vi "GUNSC_test2.vi"() -> ()   [LabVIEW 2014]
uses:
  ctest/libmap.so
  Common/Clib/lib/libmem.so.20
  expglobal.vi
  flags.vi
panel:
  in  "writekey command":string
  in  "send unsc":bool
  in  "send geom":bool
  in  "Geometry command":string
  in  "new unscrambled image":path=path "/home/ArcVIEW/Modules/GUNSC/test/ctest/test"
  in  "multiple extensions":bool=TRUE
  in  "ReadModes":u16(ring)
  in  "FPA name":string="P60"
  in  "error in (no error)":errorcluster
  in  "naxis":i32
  in  "bitpix":i32
  in  "nrows":i32
  in  "ncols":i32
  in  "scramble image on disk":path=path "/home/ArcVIEW/Modules/GUNSC/test/ctest/scr.fits"
  in  "stop":bool
  in  "Pieces":u16=1 min=1
  in  "send":bool
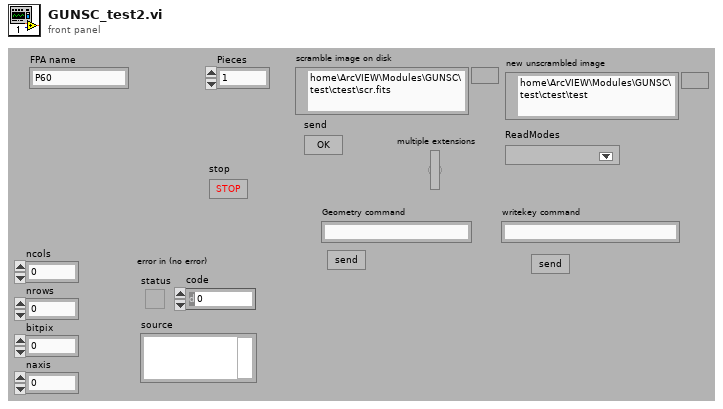
[diagram p1: front panel]
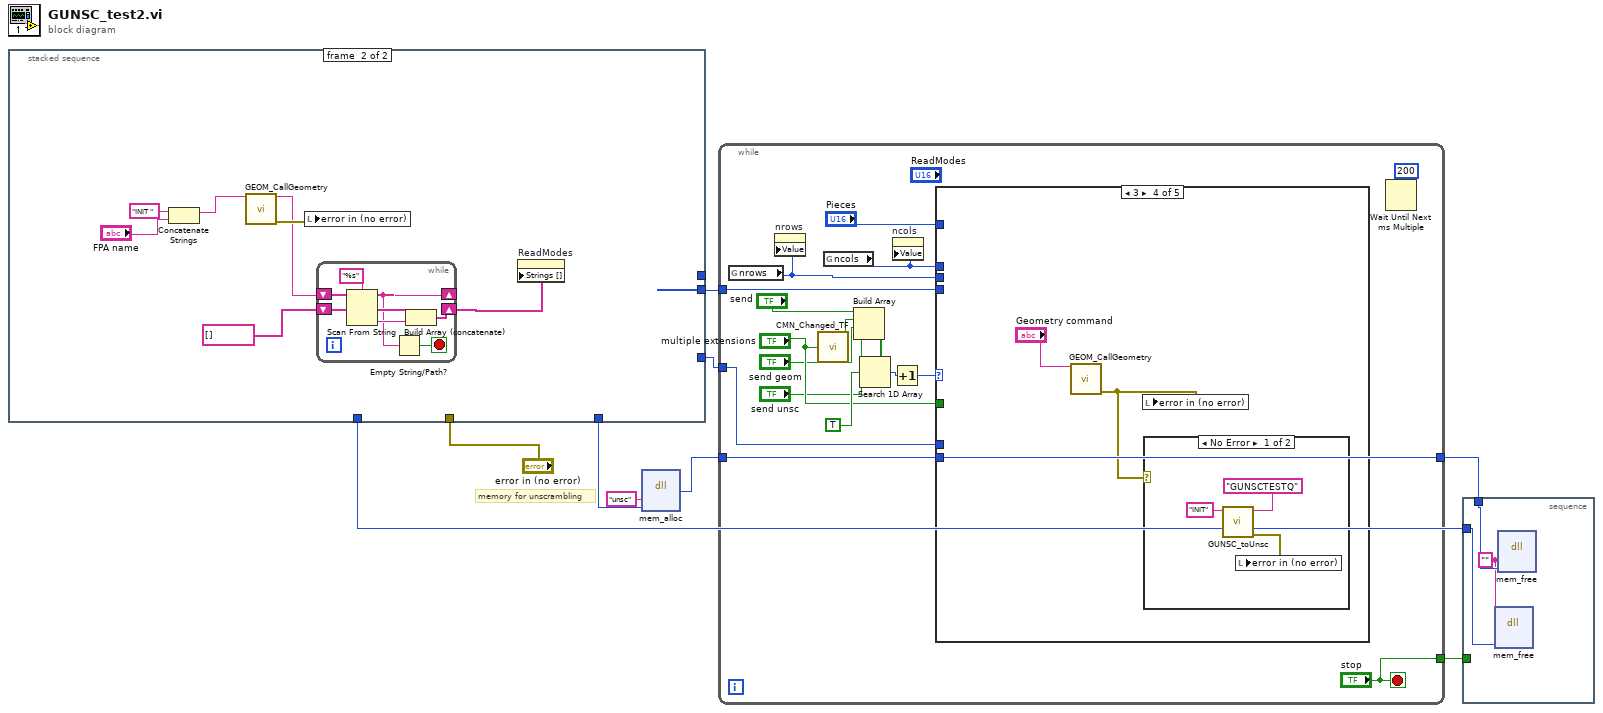
[diagram p0: block diagram]
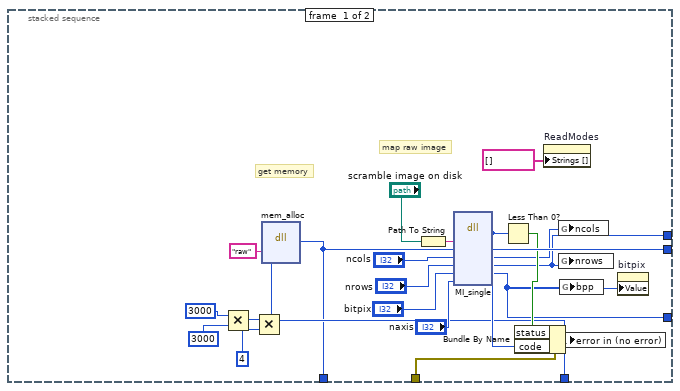
[diagram p2: hidden frame]
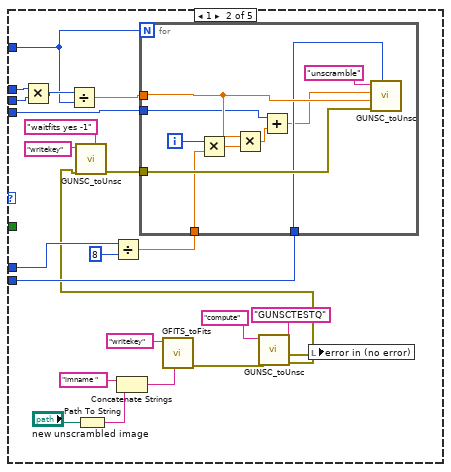
[diagram p4: hidden frame]
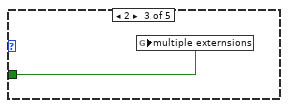
[diagram p5: hidden frame]
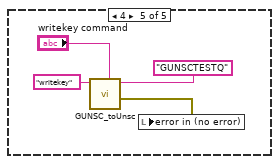
[diagram p7: hidden frame]
diagram:
  # "memory for unscrambling"
  n1 = stacked-sequence {
    tunnel: [w20 _] -> w9
    tunnel: "error in (no error)" -> [w17 _]
    tunnel: [w15 _] -> w6
    tunnel: [w12 _] -> _
    tunnel: [w11 _] -> w4
    tunnel: [w10 _] -> w1
    frame #0 {
      # "get memory"
      # "map raw image"
      n2 = Multiply(x=3000, y=3000) -> (x*y=w21:i32)
      n3 = Multiply(x=w21, y=4) -> (x*y=w15:i32)
      n4 = dll-call lib="home/sispi/Panview-1.13.0-64b/PAN/Modules/Common/Clib/lib/libmem.so.20" fn="mem_alloc"("name"="raw", "size"=w15) -> (w10:u32)  [unwired: 5 in, 2 out]
      n5 = Path To String(path="scramble image on disk") -> (string=w31:string)
      n6 = dll-call lib="uyq0/home/bonati/PAN/Modules/GUNSC/test/ctest/libmap.so" fn="MI_single"("filename"=w31, "map_addr"=w10, "ncols"="ncols", "nrows"="nrows", "bitpix"="bitpix", "naxis"="naxis") -> (w18:i32, "map_addr"=w20:u32, "ncols"=w13:i32, "nrows"=w12:i32, "bitpix"=w11:i32)  [unwired: 5 in, 2 out]
      n7 = Less Than 0?(x=w18) -> (x < 0?=w19:bool)
      n8 = Bundle By Name(cluster=w17, "status"=w19, "code"=w18) -> (w16:errorcluster)
      n9 = property on="ReadModes" class="Ring (strict)"("Strings []"=string[] []) -> ()  [unwired: 2 in, 2 out]
      n10 = global write "expglobal.vi" "ncols"(w13) -> ()
      n11 = global write "expglobal.vi" "nrows"(w12) -> ()
      n12 = global write "expglobal.vi" "bpp"(w11) -> ()
      n13 = local write "error in (no error)"(w16) -> ()
      n14 = property on="bitpix" class="DigNum (strict)"("Value"=w11) -> ()  [unwired: 2 in, 2 out]
    }
    frame #1 {
      n15 = Concatenate Strings("INIT " ("string"), "FPA name") -> (w36:string)
      n16 = call "GEOM_CallGeometry.vi"("Command"=w36) -> ("ImmedReplyString"=w33:string, "error out"=w35:errorcluster)  [unwired: 13 in]
      n17 = local write "error in (no error)"(w35) -> ()
      n18 = while {
        shift-right: [w43] -> w32
        shift-left: string[] [] -> [w42]
        shift-right: [w39] -> _
        shift-left: w33 -> [w41]
        stop <- w40 stop-if-true
        n19 = Scan From String(format string="%s", input string=w41) -> (remaining string=w39:string, output 1=w44:string)  [unwired: 3 in, 2 out]
        n20 = Empty String/Path?(string/path=w39) -> (empty?=w40:bool)
        n21 = Build Array (concatenate)(w42, w44) -> (w43:string[])
      }
      n22 = property on="ReadModes" class="Ring (strict)"("Strings []"=w32) -> ()  [unwired: 2 in, 2 out]
    }
  }
  n23 = dll-call lib="home/sispi/Panview-1.13.0-64b/PAN/Modules/Common/Clib/lib/libmem.so.20" fn="mem_alloc"("name"="unsc", "size"=w6) -> (w5:u32)  [unwired: 5 in, 2 out]
  n24 = while {
    tunnel: w9 -> [w55]
    tunnel: w5 -> [w50]
    tunnel: w4 -> [w54]
    tunnel: ["stop"] -> w3
    tunnel: [w50] -> w2
    stop <- "stop" stop-if-true
    n25 = global read "expglobal.vi" "nrows"() -> (w47:u32)
    n26 = property on="nrows" class="DigNum (strict)"("Value"=w47) -> ()  [unwired: 2 in, 2 out]
    n27 = call "CMN_Changed_TF.vi"("value"="multiple extensions") -> ("changed?"=w53:bool)  [unwired: 4 in]
    n28 = global read "expglobal.vi" "ncols"() -> (w48:u32)
    n29 = Build Array("send", w53, "send geom", "send unsc") -> (w60:bool[])
    n30 = Search 1D Array(1D array=w60, element=TRUE) -> (index of element=w58:i32)  [unwired: 1 in]
    n31 = Increment(x=w58) -> (x+1=w57:i32)
    n32 = property on="ncols" class="DigNum (strict)"("Value"=w48) -> ()  [unwired: 2 in, 2 out]
    n33 = case shown="3" w57 {
      tunnel: "Pieces" -> [_ w81 _ _ _]
      tunnel: w50 -> [_ w85 _ _ _]
      tunnel: w55 -> [_ w76 _ _ _]
      tunnel: w48 -> [_ w84 _ _ _]
      tunnel: w47 -> [_ w83 _ _ _]
      tunnel: w54 -> [_ w75 _ _ _]
      tunnel: "multiple extensions" -> [_ _ w96 _ _]
      frame 0, Default {
      }
      frame 1 {
        n34 = Multiply(x=w84, y=w83) -> (x*y=w82:u32)
        n35 = Divide(x=w82, y=w81) -> (x/y=w80:dbl)
        n36 = Path To String(path="new unscrambled image") -> (string=w65:string)
        n37 = Divide(x=w75, y=8) -> (x/y=w73:dbl)
        n38 = Concatenate Strings("imname " ("string"), w65) -> (w64:string)
        n39 = call "GFITS_toFits.vi"("key"=w64, "command"="writekey") -> ("error out"=w69:errorcluster)  [unwired: 8 in, 1 out]
        n40 = call "GUNSC_toUnsc.vi"("responseQ"="GUNSCTESTQ", "error in (no error)"=w69, "command"="compute") -> ("error out"=w63:errorcluster, "response"=w70:errorcluster)  [unwired: 7 in]
        n41 = call "GUNSC_toUnsc.vi"("key"="waitfits yes -1", "error in (no error)"=w63, "command"="writekey") -> ("error out"=w77:errorcluster)  [unwired: 7 in, 1 out]
        n42 = for {
          N: w81 -> [_]
          tunnel: w85 -> [w87]
          tunnel: w80 -> [w90]
          tunnel: w77 -> [w94]
          tunnel: w76 -> [w88]
          tunnel: w73 -> [w92]
          i -> [w93]
          n43 = Multiply(x=w93, y=w92) -> (x*y=w91:dbl)
          n44 = Multiply(x=w90, y=w91) -> (x*y=w89:dbl)
          n45 = Add(x=w88, y=w89) -> (x+y=w86:dbl)
          n46 = call "GUNSC_toUnsc.vi"("location 2"=w87, "error in (no error)"=w94, "ele Read"=w90, "location"=w86, "command"="unscramble") -> ()  [unwired: 5 in, 2 out]
        }
        n47 = local write "error in (no error)"(w70) -> ()
      }
      frame 2 {
        n48 = global write "flags.vi" "multiple externsions"(w96) -> ()
      }
      frame 3 {
        n49 = call "GEOM_CallGeometry.vi"("Command"="Geometry command") -> ("error out"=w97:errorcluster)  [unwired: 13 in, 1 out]
        n50 = local write "error in (no error)"(w97) -> ()
        n51 = case shown="No Error" w97 {
          frame No Error {
            n52 = call "GUNSC_toUnsc.vi"("responseQ"="GUNSCTESTQ", "command"="INIT") -> ("error out"=w99:errorcluster)  [unwired: 8 in, 1 out]
            n53 = local write "error in (no error)"(w99) -> ()
          }
          frame Error {
          }
        }
      }
      frame 4 {
        n54 = call "GUNSC_toUnsc.vi"("responseQ"="GUNSCTESTQ", "key"="writekey command", "command"="writekey") -> ("response"=w104:errorcluster)  [unwired: 7 in, 1 out]
        n55 = local write "error in (no error)"(w104) -> ()
      }
    }
    n56 = Wait Until Next ms Multiple(millisecond multiple=u32 200) -> ()  [unwired: 1 out]
  }
  n57 = stacked-sequence {
    tunnel: w3 -> [_]
    tunnel: w2 -> [w108]
    tunnel: w1 -> [w107]
    frame #0 {
      w106 = "" ("name")
      n58 = dll-call lib="home/sispi/Panview-1.13.0-64b/PAN/Modules/Common/Clib/lib/libmem.so.20" fn="mem_free"("name"=w106, "location"=w107) -> ()  [unwired: 6 in, 2 out]
      n59 = dll-call lib="home/sispi/Panview-1.13.0-64b/PAN/Modules/Common/Clib/lib/libmem.so.20" fn="mem_free"("name"=w106, "location"=w108) -> ()  [unwired: 6 in, 2 out]
    }
  }
